vi "AnalogDemultiplexer_NI5771.vi"() -> ()   [LabVIEW 2012]
uses:
  <vilib>/Platform/TimedLoop/XDataNode/timing_clust.ctl
  <vilib>/Platform/TimedLoop/XDataNode/nitl_modes.ctl
  <vilib>/Platform/TimedLoop/XDataNode/wakeup.ctl
  <vilib>/rvi/FIFO/Fifo_Resource/nirvififoEmulationSetSize.vi
  <vilib>/rvi/DataTransferAndStorage/Container/Common/niFpgaContainerGetUniqueNameForEmu.vi
  <vilib>/rvi/eio/common/nirviEmuTemplateMethod_errors.vi
  <vilib>/rvi/Emulation/niFpgaSctlEmulationRegisterWithScheduler.vi
  <vilib>/rvi/errors/niFpgaSetErrorForExecOnDevCompSimple.vi
  <vilib>/rvi/eio/common/nirviEmuReportErrorAndStop.vi
  <vilib>/rvi/Emulation/niFpgaSctlEmulationFifoFullMgr.vi
  <vilib>/rvi/Emulation/niFpgaSctlEmulationResourceMgr.vi
  <vilib>/rvi/Emulation/niFpgaSctlEmulationScheduler.vi
  <vilib>/rvi/Emulation/niFpgaSctlEmulationGlobalWrite.vi
  <vilib>/rvi/interface/RandomDataEmulation/nirviRandomDataFPGAFIFO.vi
  <vilib>/rvi/interface/RandomDataEmulation/niFpgaRandomDataHandleErrors.vi
  <vilib>/Platform/TimedLoop/XDataNode/XDataNode.xnode
  <vilib>/rvi/DataTransferAndStorage/Container/XNode/niFpgaContainer.xnode
  <vilib>/rvi/FIFO/Fifo_Resource/nirvififoEmulationClear.vi
  <vilib>/eio/EIONode/EIONode.xnode
  <vilib>/rvi/FIFO/Fifo_Resource/nirvififoEmulationWrite.vi
  <vilib>/rvi/FIFO/Fifo_Resource/nirvififoEmulationRead.vi
  <vilib>/rvi/interface/RandomDataEmulation/nirviRandomDataFpgaReadWriteTemplate.vi
  <vilib>/Platform/TimedLoop/XDataNode/XDNodeRunTimeDep.lvlib
panel:
  in  "BaselineU8 Ch2":u8
  in  "BaselineU8 Ch1":u8
  out "InterloopFIFO timeout":bool
  in  "Clear Interloop FIFO":bool
  out "Pixel counter A2":u32
  out "ToHost FIFO Overflow A2":bool
  out "Pixel counter A1":u32
  out "ToHost FIFO Overflow A1":bool
  out "Acquiring":bool
  in  "Wait for trigger":bool
  in  "Acquire":bool
  in  "Requested pixels A2":u32=100000 caption="Requested pixels"
  in  "Acquire continuously":bool=TRUE
  in  "Requested pixels A1":u32=100000 caption="Requested pixels"
  in  "Samples per pixel Acq A2":u16=10000 caption="Samples per pixel Acq"
  in  "Samples per pixel Acq A1":u16=10000 caption="Samples per pixel Acq"
  in  "Samples per pixel A2":u16=10000
  in  "Samples per pixel A1":u16=10000
  out "InterloopFIFO overflow":bool
  out "IO Module\\AI Over Range":bool
  in  "User Command Commit":bool
  in  "User Command":u8
  out "User Command Idle":bool
  out "User Command Status":u8
  in  "User Data 0":u16
  in  "User Data 1":u8
  out "PLL Locked":bool
  out "User Error":bool
  out "Configured?":bool
  # "5771 IO module configuration"
  # "Analog demultiplexer"
  # "Acquisition control"
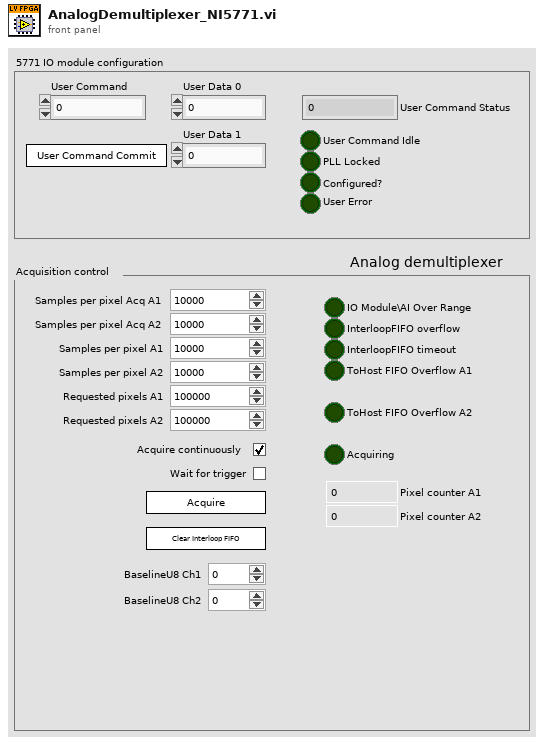
[diagram p1: front panel]
types:
  T1 = typedef "XDNodeRunTimeDep.lvlib/timing_clust.ctl" = cluster{"Expected End [f-1]":u64, "Actual End [f-1]":u64, "Finished Late? [f-1]":bool, "Expected End [i-1]":u64, "Actual End [i-1]":u64, "Finished Late? [i-1]":bool, "Expected Start [i]":u64, "Actual Start [i]":u64, "Expected Start [f]":u64, "Actual Start [f]":u64, "Source Name":string, "Structure Name":string, "Period":i64, "Deadline":i64, "Offset":i64, "Start":i64, "Priority":i32, "Timeout":i32, "Mode":T2, "Wakeup Reason":T3, "Error":errorcluster, "Source Type":string, "Secondary Source Type":string, "Global End Time":u64, "Global Start Time":u64, "Frame Duration":u64, "Iteration Duration":u64, "Assigned CPU":i32, "I/O Scan Engine Mode":u32}
  T2 = typedef "XDNodeRunTimeDep.lvlib/nitl_modes.ctl" = enum32{"No Change", "Process missed periods, maintain original phase", "Discard missed periods, maintain original phase", "Process missed periods, ignore original phase", "Discard missed periods, ignore original phase"}
  T3 = typedef "XDNodeRunTimeDep.lvlib/wakeup.ctl" = enum32{"Normal", "Aborted", "Asynchronous wakeup", "Timing source error", "Timed loop error", "Timeout"}
  T4 = cluster{"IO Module\\AI 0 Data N-7":u8, "IO Module\\AI 0 Data N-6":u8, "IO Module\\AI 0 Data N-5":u8, "IO Module\\AI 0 Data N-4":u8, "IO Module\\AI 0 Data N-3":u8, "IO Module\\AI 0 Data N-2":u8, "IO Module\\AI 0 Data N-1":u8, "IO Module\\AI 0 Data N":u8, "IO Module\\Synchronous Trigger Input":u8}
  T5 = cluster{"IO Module\\AI 1 Data N-7":u8, "IO Module\\AI 1 Data N-6":u8, "IO Module\\AI 1 Data N-5":u8, "IO Module\\AI 1 Data N-4":u8, "IO Module\\AI 1 Data N-3":u8, "IO Module\\AI 1 Data N-2":u8, "IO Module\\AI 1 Data N-1":u8, "IO Module\\AI 1 Data N":u8, "IO Module\\Synchronous Trigger Input":u8}
  T6 = cluster{"Data A1 out":u64, "Data A1 out":u64, "Data A2 out":u64, "Data A2 out":u64}
  T7 = cluster{"A1Ch1":u64, "A1Ch2":u64, "A2Ch1":u64, "A2Ch2":u64}
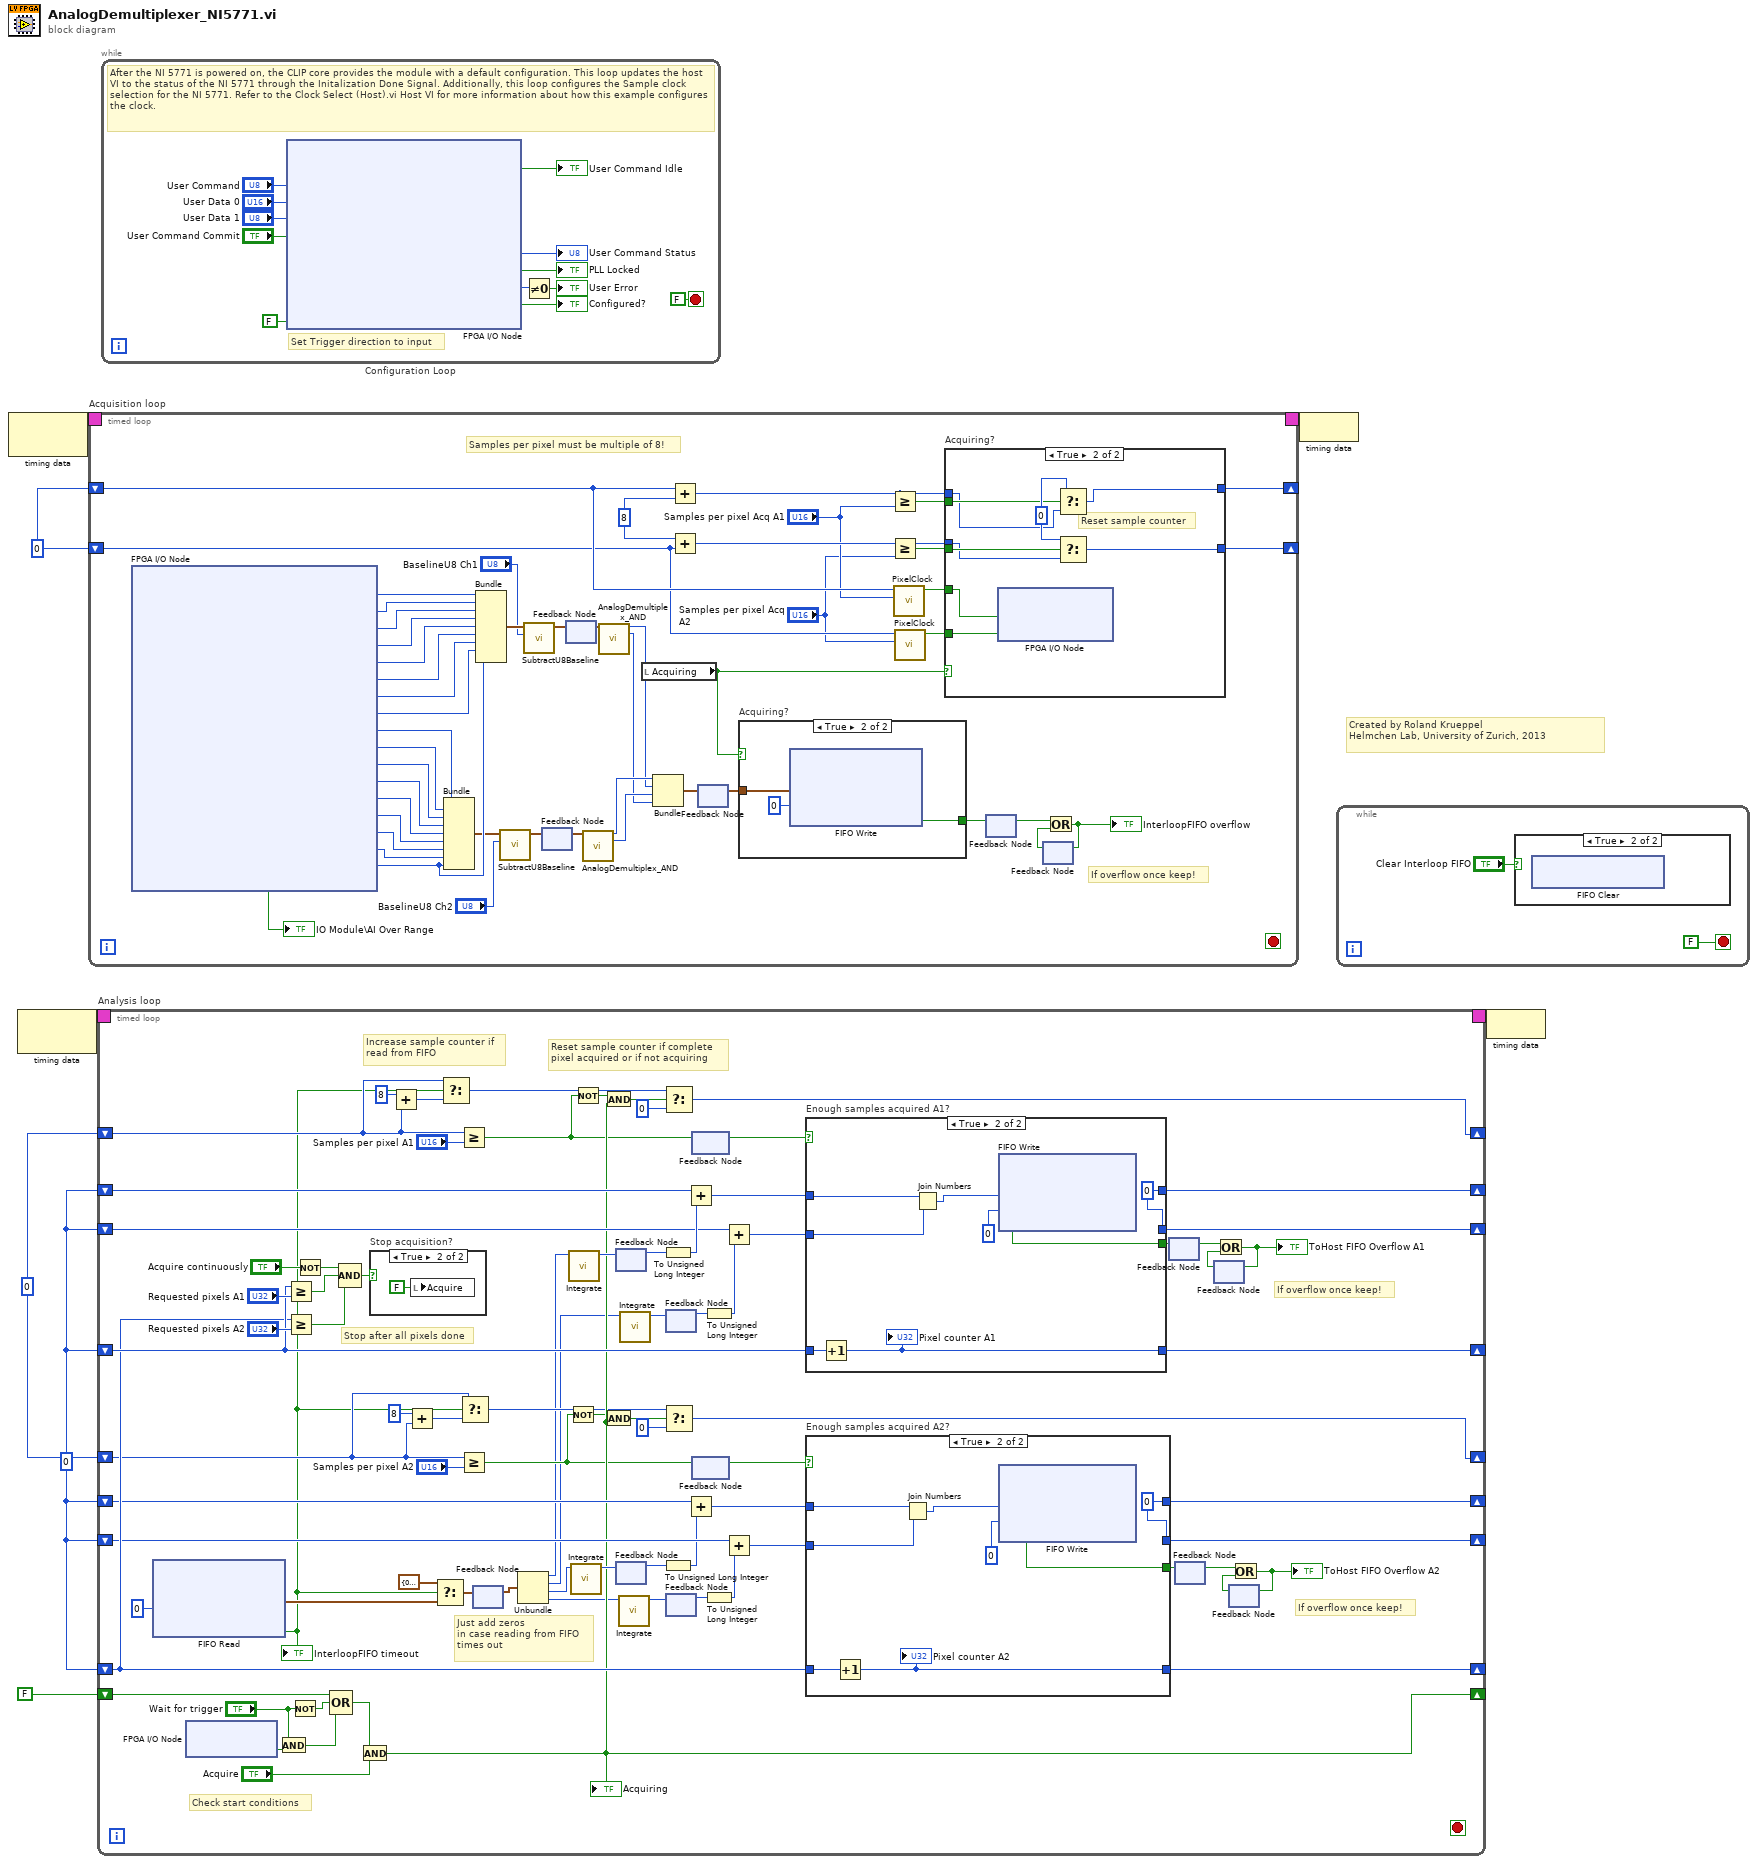
[diagram p0: block diagram]
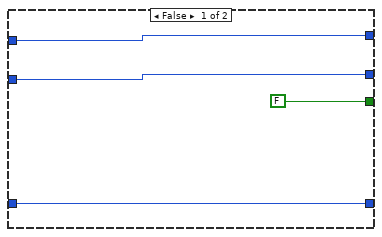
[diagram p3: hidden frame]
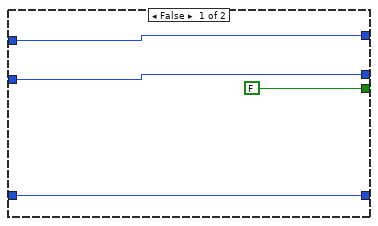
[diagram p4: hidden frame]
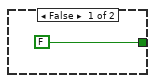
[diagram p6: hidden frame]
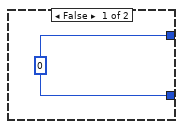
[diagram p7: hidden frame]
diagram:
  w2 = u16 0
  w1 = u32 0 ("Integrator out")
  w4 = u16 0
  # "Created by Roland Krueppel\nHelmchen Lab, University of Zurich, 2013"
  n1 = node-c288() -> (w8:T1)  [unwired: 1 in]
  n2 = node-c288() -> (w6:T1)  [unwired: 1 in]
  n3 = timed-loop "Acquisition loop" {
    timing: w8 -> [_]
    timing-out: [_] -> w7
    shift-right: [w36] -> _
    shift-left: w4 -> [w11]
    shift-right: [w37] -> _
    shift-left: w4 -> [w14]
    stop <- _ stop-if-true
    w31 = u16 8 ("y")
    # "If overflow once keep!"
    # "Samples per pixel must be multiple of 8!"
    n4 = xnode "FPGA I/O Node"() -> ("IO Module\\AI 1 Data N-7"=w50:u8, "IO Module\\AI 1 Data N-6"=w49:u8, "IO Module\\AI 1 Data N-5"=w48:u8, "IO Module\\AI 1 Data N-4"=w47:u8, "IO Module\\AI 1 Data N-3"=w46:u8, "IO Module\\AI 1 Data N-2"=w45:u8, "IO Module\\AI 1 Data N-1"=w44:u8, "IO Module\\AI 1 Data N"=w43:u8, "IO Module\\AI 0 Data N-7"=w51:u8, "IO Module\\AI 0 Data N-6"=w52:u8, "IO Module\\AI 0 Data N-5"=w53:u8, "IO Module\\AI 0 Data N-4"=w54:u8, "IO Module\\AI 0 Data N-3"=w55:u8, "IO Module\\AI 0 Data N-2"=w56:u8, "IO Module\\AI 0 Data N-1"=w57:u8, "IO Module\\AI 0 Data N"=w58:u8, "IO Module\\Synchronous Trigger Input"=w38:u8, "IO Module\\AI Over Range"=→"IO Module\\AI Over Range":bool)  [unwired: 18 in, 18 out]
    n5 = Bundle("IO Module\\AI 0 Data N-7"=w51, "IO Module\\AI 0 Data N-6"=w52, "IO Module\\AI 0 Data N-5"=w53, "IO Module\\AI 0 Data N-4"=w54, "IO Module\\AI 0 Data N-3"=w55, "IO Module\\AI 0 Data N-2"=w56, "IO Module\\AI 0 Data N-1"=w57, "IO Module\\AI 0 Data N"=w58, "IO Module\\Synchronous Trigger Input"=w38) -> (w18:T4)  [unwired: 1 in]
    n6 = Bundle("IO Module\\AI 1 Data N-7"=w50, "IO Module\\AI 1 Data N-6"=w49, "IO Module\\AI 1 Data N-5"=w48, "IO Module\\AI 1 Data N-4"=w47, "IO Module\\AI 1 Data N-3"=w46, "IO Module\\AI 1 Data N-2"=w45, "IO Module\\AI 1 Data N-1"=w44, "IO Module\\AI 1 Data N"=w43, "IO Module\\Synchronous Trigger Input"=w38) -> (w21:T5)  [unwired: 1 in]
    n7 = call "SubtractU8Baseline.vi"("Baseline U8"="BaselineU8 Ch2", "Analog data cluster in"=w18) -> ("Analog data cluster out"=w17:T4)  [unwired: 9 in]
    n8 = call "SubtractU8Baseline.vi"("Baseline U8"="BaselineU8 Ch1", "Analog data cluster in"=w21) -> ("Analog data cluster out"=w20:T4)  [unwired: 9 in]
    n9 = feedback #1() -> (w22:T4)  [unwired: 1 in]
    n10 = feedback-in #1(w17) -> ()
    n11 = feedback-in #2(w20) -> ()
    n12 = feedback #2() -> (w34:T4)  [unwired: 1 in]
    n13 = call "AnalogDemultiplex_AND.vi"("Analog data cluster"=w22) -> ("Data A1 out"=w42:u64, "Data A2 out"=w40:u64)  [unwired: 13 in]
    n14 = call "AnalogDemultiplex_AND.vi"("Analog data cluster"=w34) -> ("Data A1 out"=w41:u64, "Data A2 out"=w39:u64)  [unwired: 13 in]
    n15 = local read "Acquiring"() -> (w35:bool)
    n16 = Bundle("Data A1 out"=w42, "Data A1 out"=w41, "Data A2 out"=w40, "Data A2 out"=w39) -> (w33:T6)  [unwired: 1 in]
    n17 = Add(x=w14, y=w31) -> (x+y=w29:u16)
    n18 = Add(x=w31, y=w11) -> (x+y=w30:u16)
    n19 = feedback #3() -> (w32:T6)  [unwired: 1 in]
    n20 = feedback-in #3(w33) -> ()
    n21 = case "Acquiring?" shown="True" w35 {
      tunnel: w32 -> [_ w61]
      tunnel: [FALSE ("Timed Out?") w60] -> w24
      frame False {
      }
      frame True {
        n22 = xnode ("FIFO Write")("Element"=w61, "Timeout"=0) -> ("Timed Out?"=w60:bool)  [unwired: 1 in, 1 out]
      }
    }
    n23 = Greater Or Equal?(x=w29, y="Samples per pixel Acq A1") -> (x >= y?=w28:bool)
    n24 = Greater Or Equal?(x=w30, y="Samples per pixel Acq A2") -> (x >= y?=w27:bool)
    n25 = call "PixelClock.vi"("Samples per pixel"="Samples per pixel Acq A1", "Sample counter"=w14) -> ("Pixel clock"=w12:bool)  [unwired: 9 in]
    n26 = call "PixelClock.vi"("Samples per pixel"="Samples per pixel Acq A2", "Sample counter"=w11) -> ("Pixel clock"=w9:bool)  [unwired: 9 in]
    n27 = case "Acquiring?" shown="True" w35 {
      tunnel: w30 -> [_ w65]
      tunnel: w29 -> [_ w67]
      tunnel: [w63 w71] -> w37
      tunnel: [w63 w70] -> w36
      tunnel: w28 -> [_ w68]
      tunnel: w12 -> [_ w64]
      tunnel: w9 -> [_ w69]
      tunnel: w27 -> [_ w66]
      frame False {
        w63 = u16 0 ("t")
      }
      frame True {
        w72 = u16 0 ("t")
        # "Reset sample counter"
        n28 = xnode "FPGA I/O Node"("Pixel clock"=w64, "Pixel clock A2"=w69) -> ()  [unwired: 2 in, 2 out]
        n29 = Select(t=w72, s=w68, f=w67) -> (s? t:f=w71:u16)
        n30 = Select(t=w72, s=w66, f=w65) -> (s? t:f=w70:u16)
      }
    }
    n31 = feedback-in #4(w24) -> ()
    n32 = feedback #4() -> (w23:bool)  [unwired: 1 in]
    n33 = feedback #5() -> (w25:bool)  [unwired: 1 in]
    n34 = Or(x=w23, y=w25) -> (x .or. y?=w26:bool)
    "InterloopFIFO overflow" <- w26
    n35 = feedback-in #5(w26) -> ()
  }
  n36 = timed-loop "Analysis loop" {
    timing: w6 -> [_]
    timing-out: [_] -> w5
    shift-right: [w104] -> _
    shift-left: w2 -> [w92]
    shift-right: [w94] -> _
    shift-left: w2 -> [w95]
    shift-right: [w155] -> _
    shift-left: w1 -> [w121]
    shift-right: [w156] -> _
    shift-left: w1 -> [w116]
    shift-right: [w90] -> _
    shift-left: FALSE -> [w142]
    shift-right: [w141] -> _
    shift-left: w1 -> [w137]
    shift-right: [w140] -> _
    shift-left: w1 -> [w114]
    shift-right: [w139] -> _
    shift-left: w1 -> [w115]
    shift-right: [w138] -> _
    shift-left: w1 -> [w136]
    stop <- _ stop-if-true
    # "Just add zeros\nin case reading from FIFO\ntimes out"
    # "Stop after all pixels done"
    # "Increase sample counter if\nread from FIFO"
    # "Reset sample counter if complete\npixel acquired or if not acquiring"
    # "If overflow once keep!"
    # "If overflow once keep!"
    # "Check start conditions"
    n37 = xnode ("FIFO Read")("Timeout"=0) -> ("Element"=w98:T7, "Timed Out?"=w91:bool)  [unwired: 1 in, 1 out]
    "InterloopFIFO timeout" <- w91
    n38 = xnode "FPGA I/O Node"() -> ("TriggerIn"=w147:bool)  [unwired: 1 in, 1 out]
    n39 = And(x="Wait for trigger", y=w147) -> (x .and. y?=w144:bool)
    n40 = Greater Or Equal?(x=w137, y="Requested pixels A1") -> (x >= y?=w150:bool)
    n41 = Greater Or Equal?(x=w136, y="Requested pixels A2") -> (x >= y?=w149:bool)
    n42 = Not(x="Wait for trigger") -> (.not. x?=w145:bool)
    n43 = Not(x="Acquire continuously") -> (.not. x?=w151:bool)
    n44 = Compound Arithmetic op=OR(w142, w145, w144) -> (w143:bool)
    n45 = Compound Arithmetic op=AND(w151, w150, w149) -> (w135:bool)
    n46 = And(x=w143, y="Acquire") -> (x .and. y?=w90:bool)
    "Acquiring" <- w90
    n47 = case "Stop acquisition?" shown="True" w135 {
      frame False {
      }
      frame True {
        n48 = local write "Acquire"(FALSE ("Acquire")) -> ()
      }
    }
    n49 = Add(x=u16 8, y=w92) -> (x+y=w93:u16)
    n50 = Add(x=u16 8, y=w95) -> (x+y=w96:u16)
    n51 = Select(t=T7 {"A1Ch1"=0, "A1Ch2"=0, "A2Ch1"=0, "A2Ch2"=0}, s=w91, f=w98) -> (s? t:f=w99:T7)
    n52 = Select(t=w92, s=w91, f=w93) -> (s? t:f=w80:u16)
    n53 = Greater Or Equal?(x=w92, y="Samples per pixel A1") -> (x >= y?=w85:bool)
    n54 = Greater Or Equal?(x=w95, y="Samples per pixel A2") -> (x >= y?=w88:bool)
    n55 = Select(t=w95, s=w91, f=w96) -> (s? t:f=w82:u16)
    n56 = feedback-in #6(w99) -> ()
    n57 = feedback #6() -> (w124:T7)  [unwired: 1 in]
    n58 = Unbundle(w124) -> ("A1Ch1"=w79:u64, "A1Ch2"=w78:u64, "A2Ch1"=w77:u64, "A2Ch2"=w76:u64)
    n59 = Not(x=w88) -> (.not. x?=w89:bool)
    n60 = call "Integrate.vi"("New samples in"=w79) -> ("Sum out"=w123:u16)  [unwired: 10 in]
    n61 = call "Integrate.vi"("New samples in"=w77) -> ("Sum out"=w118:u16)  [unwired: 10 in]
    n62 = Not(x=w85) -> (.not. x?=w86:bool)
    n63 = And(x=w86, y=w90) -> (x .and. y?=w84:bool)
    n64 = And(x=w89, y=w90) -> (x .and. y?=w87:bool)
    n65 = feedback-in #7(w123) -> ()
    n66 = feedback #7() -> (w120:u16)  [unwired: 1 in]
    n67 = feedback #8() -> (w117:u16)  [unwired: 1 in]
    n68 = feedback-in #8(w118) -> ()
    n69 = call "Integrate.vi"("New samples in"=w76) -> ("Sum out"=w112:u16)  [unwired: 10 in]
    n70 = call "Integrate.vi"("New samples in"=w78) -> ("Sum out"=w109:u16)  [unwired: 10 in]
    n71 = To Unsigned Long Integer(number=w120) -> (unsigned 32bit integer=w119:u32)
    n72 = To Unsigned Long Integer(number=w117) -> (unsigned 32bit integer=w113:u32)
    n73 = Select(t=w80, s=w84, f=u16 0 ("t")) -> (s? t:f=w104:u16)
    n74 = Select(t=w82, s=w87, f=u16 0) -> (s? t:f=w94:u16)
    n75 = feedback #9() -> (w108:u16)  [unwired: 1 in]
    n76 = feedback-in #9(w109) -> ()
    n77 = feedback #10() -> (w111:u16)  [unwired: 1 in]
    n78 = feedback-in #10(w112) -> ()
    n79 = Add(x=w121, y=w119) -> (x+y=w101:u32)
    n80 = Add(x=w116, y=w113) -> (x+y=w103:u32)
    n81 = feedback #11() -> (w106:bool)  [unwired: 1 in]
    n82 = feedback-in #11(w85) -> ()
    n83 = feedback #12() -> (w105:bool)  [unwired: 1 in]
    n84 = feedback-in #12(w88) -> ()
    n85 = To Unsigned Long Integer(number=w108) -> (unsigned 32bit integer=w107:u32)
    n86 = To Unsigned Long Integer(number=w111) -> (unsigned 32bit integer=w110:u32)
    n87 = Add(x=w114, y=w107) -> (x+y=w100:u32)
    n88 = Add(x=w115, y=w110) -> (x+y=w102:u32)
    n89 = case "Enough samples acquired A1?" shown="True" w106 {
      tunnel: [w172 w180] -> w155
      tunnel: w137 -> [w173 w176]
      tunnel: [w173 w181] -> w141
      tunnel: [w171 w180] -> w140
      tunnel: w101 -> [w172 w175]
      tunnel: w100 -> [w171 w174]
      tunnel: [FALSE ("Timed Out?") w179] -> w130
      frame False {
      }
      frame True {
        w180 = u32 0 ("Integrator out")
        n90 = Increment(x=w176) -> (x+1=w181:u32)
        "Pixel counter A1" <- w181
        n91 = Join Numbers(hi=w175, lo=w174) -> ((hi.lo)=w177:u64)
        n92 = xnode ("FIFO Write")("Element"=w177, "Timeout"=0) -> ("Timed Out?"=w179:bool)  [unwired: 1 in, 1 out]
      }
    }
    n93 = case "Enough samples acquired A2?" shown="True" w105 {
      tunnel: [w160 w169] -> w156
      tunnel: [w159 w169] -> w139
      tunnel: w136 -> [w161 w164]
      tunnel: [w161 w168] -> w138
      tunnel: w103 -> [w160 w163]
      tunnel: w102 -> [w159 w162]
      tunnel: [FALSE ("Timed Out?") w167] -> w126
      frame False {
      }
      frame True {
        w169 = u32 0 ("Integrator out")
        n94 = Increment(x=w164) -> (x+1=w168:u32)
        "Pixel counter A2" <- w168
        n95 = Join Numbers(hi=w163, lo=w162) -> ((hi.lo)=w165:u64)
        n96 = xnode ("FIFO Write")("Element"=w165, "Timeout"=0) -> ("Timed Out?"=w167:bool)  [unwired: 1 in, 1 out]
      }
    }
    n97 = feedback-in #13(w130) -> ()
    n98 = feedback #13() -> (w129:bool)  [unwired: 1 in]
    n99 = feedback #14() -> (w125:bool)  [unwired: 1 in]
    n100 = feedback-in #14(w126) -> ()
    n101 = feedback #15() -> (w131:bool)  [unwired: 1 in]
    n102 = Or(x=w129, y=w131) -> (x .or. y?=w132:bool)
    "ToHost FIFO Overflow A1" <- w132
    n103 = feedback-in #15(w132) -> ()
    n104 = feedback #16() -> (w127:bool)  [unwired: 1 in]
    n105 = Or(x=w125, y=w127) -> (x .or. y?=w128:bool)
    "ToHost FIFO Overflow A2" <- w128
    n106 = feedback-in #16(w128) -> ()
  }
  n107 = while "Configuration Loop" {
    stop <- FALSE stop-if-true
    # "Set Trigger direction to input"
    # "After the NI 5771 is powered on, the CLIP core provides the module with a default configuration. This loop updates the host VI to the status of the NI 5771 through the Initalization Done Signal. Additionally, this loop configures the Sample clock selection for the NI 5771. Refer to the Clock Select (Host).vi Host VI for more information about how this example configures the clock."
    n108 = xnode "FPGA I/O Node"("IO Module\\User Command"="User Command", "IO Module\\User Data 0"="User Data 0", "IO Module\\User Data 1"="User Data 1", "IO Module\\User Command Commit"="User Command Commit", "IO Module\\Trigger WE"=FALSE ("IO Module\\Trigger WE")) -> ("IO Module\\User Command Idle"=→"User Command Idle":bool, "IO Module\\User Command Status"=→"User Command Status":u8, "IO Module\\PLL Locked"=→"PLL Locked":bool, "IO Module\\User Error"=w189:u8, "IO Module\\Initialization Done"=→"Configured?":bool)  [unwired: 10 in, 10 out]
    n109 = Not Equal To 0?(x=w189) -> (x != 0?=→"User Error":bool)
  }
  n110 = node-c288(w7) -> ()
  n111 = while {
    stop <- FALSE stop-if-true
    n112 = case shown="True" "Clear Interloop FIFO" {
      frame False {
      }
      frame True {
        n113 = xnode ("FIFO Clear")() -> ()  [unwired: 1 in, 1 out]
      }
    }
  }
  n114 = node-c288(w5) -> ()
